vi "FTW-Test-JSON-Units.vi"() -> (0 "Test Result":errorcluster)   [LabVIEW 2015]
uses:
  src/json/core/FTW-JSON-Core-Type.ctl
  src/reflection/FTW-Reflection-Types.ctl
  src/json/FTW-JSON-Construct-FromBuffer.vi
  lib/FTW-KernelFilepath.vi
  codegen/xnode/json/fetch/FTW-JSON-Core-GetFlattenedValue.vi
  src/error/FTW-ERR-ThrowInvalidReferenceError.vi
  src/json/core/FTW-JSON-Core-ElementType.vi
  src/json/FTW-JSON-SerializeAndDestroy.vi
  codegen/xnode/FTW-JSON-Fetch.xnode
  src/json/FTW-JSON-Type.ctl
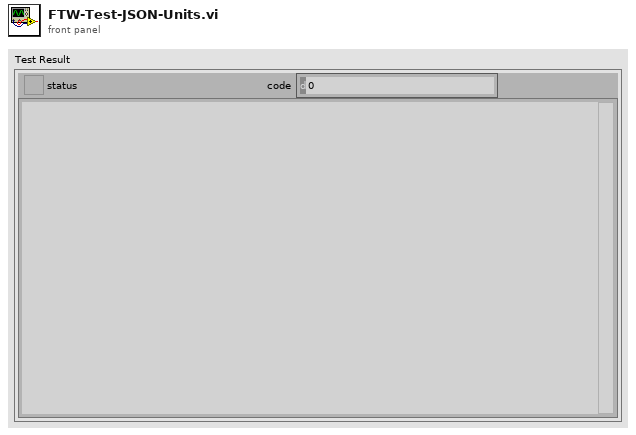
[diagram p1: front panel]
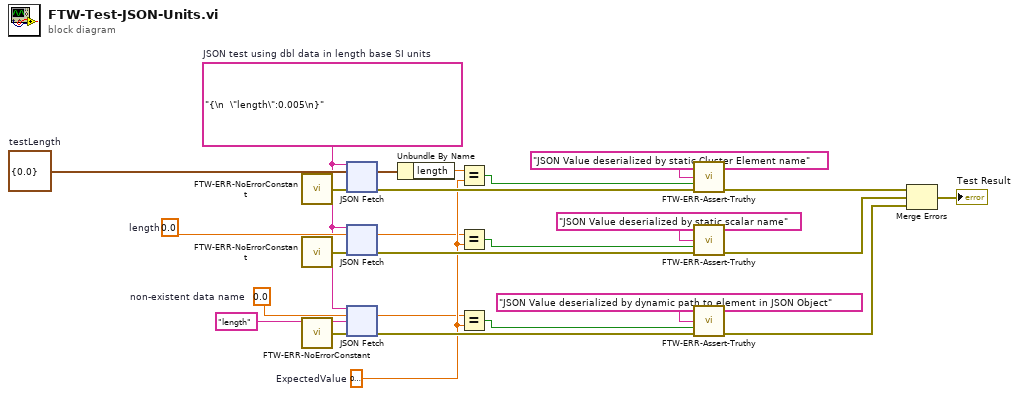
[diagram p0: block diagram]
diagram:
  w4 = dbl[unit] 0.0  # non-existent data name
  w10 = dbl[unit] 0.005  # ExpectedValue
  w5 = dbl[unit] 0.0  # length
  w7 = cluster{"length":dbl[unit]} {"length"=0.0}  # testLength
  w2 = "{\n  \"length\":0.005\n}"  # JSON test using dbl data in length base SI units
  n1 = call "FTW-ERR-NoErrorConstant.vi"() -> ("no error"=w26:errorcluster)
  n2 = call "FTW-ERR-NoErrorConstant.vi"() -> ("no error"=w25:errorcluster)
  n3 = call "FTW-ERR-NoErrorConstant.vi"() -> ("no error"=w9:errorcluster)
  n4 = xnode "JSON Fetch"("JSON"=w2, "Element Type and Default Value"=w7, "error in"=w26) -> ("Value"=w6:cluster{"length":dbl[unit]}, "error out"=w16:errorcluster)  [unwired: 2 in, 3 out]
  n5 = xnode "JSON Fetch"("JSON"=w2, "Element Type and Default Value"=w5, "error in"=w25) -> ("Value"=w1:dbl[unit], "error out"=w19:errorcluster)  [unwired: 2 in, 3 out]
  n6 = xnode "JSON Fetch"("JSON"=w2, "Element Type and Default Value"=w4, "Element Path"="length", "error in"=w9) -> ("Value"=w3:dbl[unit], "error out"=w23:errorcluster)  [unwired: 1 in, 3 out]
  n7 = Unbundle By Name(w6) -> ("length"=w24:dbl[unit])
  n8 = Equal?(x=w24, y=w10) -> (x = y?=w17:bool)
  n9 = Equal?(x=w1, y=w10) -> (x = y?=w20:bool)
  n10 = Equal?(x=w3, y=w10) -> (x = y?=w21:bool)
  n11 = call "FTW-ERR-Assert-Truthy.vi"("Assertion"="JSON Value deserialized by static Cluster Element name", "Assertion holds true?"=w17, "error in"=w16) -> ("error out"=w15:errorcluster)  [unwired: 12 in]
  n12 = call "FTW-ERR-Assert-Truthy.vi"("Assertion"="JSON Value deserialized by static scalar name", "Assertion holds true?"=w20, "error in"=w19) -> ("error out"=w18:errorcluster)  [unwired: 12 in]
  n13 = call "FTW-ERR-Assert-Truthy.vi"("Assertion"="JSON Value deserialized by dynamic path to element in JSON Object", "Assertion holds true?"=w21, "error in"=w23) -> ("error out"=w22:errorcluster)  [unwired: 12 in]
  n14 = Merge Errors(w15, w18, w22) -> (→"Test Result":errorcluster)
